vi "CalcTheta.vi"() -> (3 "ThetaValues":dbl[](array[numeric]))   [LabVIEW 2018]
panel:
  # "Front of bot"
  # "L"
  # "W"
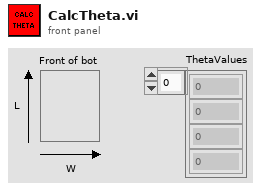
[diagram p1: front panel]
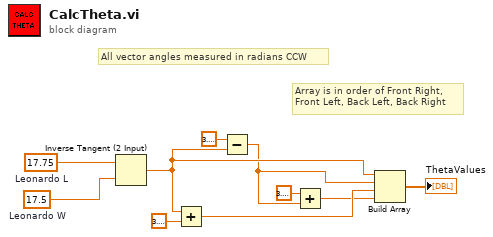
[diagram p0: block diagram]
diagram:
  w6 = 17.5  # Leonardo W
  w7 = 17.75  # Leonardo L
  # "Array is in order of Front Right,\nFront Left, Back Left, Back Right"
  # "All vector angles measured in radians CCW"
  n1 = Inverse Tangent (2 Input)(1:w6, 2:w7) -> (0:w4:dbl)
  n2 = Add(x=w4, y=3.141592653589793) -> (x+y=w2:dbl)
  n3 = Subtract(x=3.141592653589793, y=w4) -> (x-y=w3:dbl)
  n4 = Add(x=3.141592653589793, y=w3) -> (x+y=w1:dbl)
  n5 = Build Array(w4, w3, w2, w1) -> (→"ThetaValues":dbl[])
